vi "Zombie Left Cell String.vi"(8 "Error In":errorcluster, 10 "Bookmark ID":u32, 11 "VI Path":path) -> (0 "Error Out":errorcluster, 3 "Text":string)   [LabVIEW 2017, in "Graveyard.lvlib"]
doc: "Gets the left cell string for a zombie child item in the bookmarks tree. If the Spirit frame is enabled, then the text is \"Corpse\". If the Corpse frame is enabled, then the text is \"Reanimated\"."
uses:
  Graveyard.lvlib
  Eulogy/Public/Typedefs/Zombie States.ctl
  Eulogy/Eulogy.lvlib
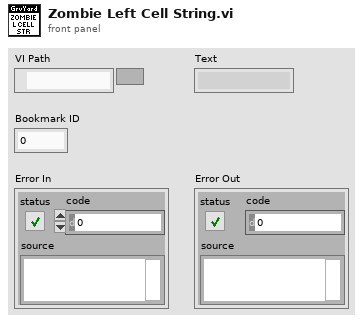
[diagram p1: front panel]
types:
  T1 = typedef "Eulogy.lvlib/Zombie States.ctl" = enum16{"Corpse", "Reanimated"}
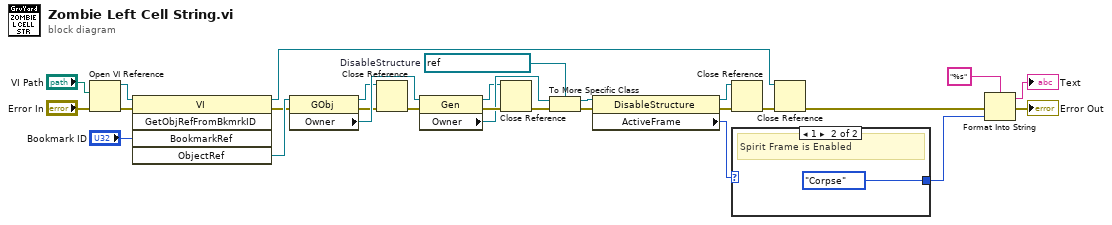
[diagram p0: block diagram]
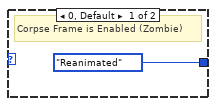
[diagram p2: hidden frame]
diagram:
  w22 = refnum<vi> refnum  # DisableStructure
  n1 = Open VI Reference(vi path="VI Path", error in (no error)="Error In") -> (vi reference=w23:refnum<vi>, error out=w24:errorcluster)  [unwired: 4 in]
  n2 = invoke class="VI" method="GetObjRefFromBkmrkID"(reference=w23, error in=w24, "BookmarkRef"="Bookmark ID") -> (reference out=w14:refnum<vi>, error out=w5:errorcluster, "ObjectRef"=w28:refnum<vi>)  [unwired: 2 in, 2 out]
  n3 = property class="GObj"(reference=w28, error in=w5) -> (reference out=w11:refnum<vi>, error out=w12:errorcluster, "Owner"=w16:refnum<vi>)
  n4 = Close Reference(reference=w11, error in (no error)=w12) -> (error out=w10:errorcluster)
  n5 = property class="Gen"(reference=w16, error in=w10) -> (reference out=w6:refnum<vi>, error out=w9:errorcluster, "Owner"=w8:refnum<vi>)
  n6 = Close Reference(reference=w6, error in (no error)=w9) -> (error out=w7:errorcluster)
  n7 = To More Specific Class(target class=w22, reference=w8, error in=w7) -> (specific class reference=w21:refnum<vi>, error out=w20:errorcluster)
  n8 = property class="DisableStructure"(reference=w21, error in=w20) -> (reference out=w17:refnum<vi>, error out=w18:errorcluster, "ActiveFrame"=w19:i16)
  n9 = Close Reference(reference=w17, error in (no error)=w18) -> (error out=w13:errorcluster)
  n10 = case shown="1" w19 {
    tunnel: [Zombie_States."Reanimated" ("Zombie State") Zombie_States."Corpse" ("Zombie State")] -> w3
    frame 0, Default {
      # "Corpse Frame is Enabled (Zombie)"
    }
    frame 1 {
      # "Spirit Frame is Enabled"
    }
  }
  n11 = Close Reference(reference=w14, error in (no error)=w13) -> (error out=w15:errorcluster)
  n12 = Format Into String(format string="%s", error in=w15, w3) -> (resulting string=→"Text":string, error out=→"Error Out":errorcluster)  [unwired: 1 in]
